vi "RT_Example.vi"() -> ()   [LabVIEW 2014]
uses:
  <vilib>/NI/cRIO Wfm/ChannelConfig.ctl
  <vilib>/FPGAPlugInAG/sbRIO-9651/niLvFpga_Open_sbRIO-9651.vi
  <vilib>/rvi/interface/common/dynamic/niFpgaDynamicAddResources.vi
  <vilib>/FPGAPlugInAG/Dynamic/niLvFpga_Reset_Dynamic.vi
  <vilib>/FPGAPlugInAG/Dynamic/niLvFpga_Run_Dynamic.vi
  <vilib>/NI/cRIO Wfm/AcqRead(Wfm).vi
  <vilib>/measure/matone.llb/Extract Single Tone Information 1 Chan.vi
  <vilib>/FPGAPlugInAG/Dynamic/niLvFpga_Close_Dynamic.vi
  <vilib>/rvi/interface/nirviOpenFPGA/nirviOpenFPGA.xnode
  FPGA Bitfiles/FPGAMainScripted.lvbitx
  <vilib>/rvi/interface/nirviMethod/nirviMethod.xnode
  <vilib>/rvi/interface/nirviCloseFPGA/nirviCloseFPGA.xnode
  <vilib>/NI/cRIO Wfm/cRIO Wfm.lvlib
  <vilib>/measure/NI_MAPro.lvlib
  <vilib>/rvi/interface/nirviReadWriteControl/nirviReadWriteControl.xnode
  NiFpgaLv.dll
  <vilib>/Utility/error.llb/Error Cluster From Error Code.vi
  <vilib>/rvi/interface/Simulation/niFpgaSimulationCallBeginRW.vi
  <vilib>/rvi/errors/niLvFpgaAdjustHostInterfaceError.vi
panel:
  out "Samples Remaining":u32
  out "Detected Amplitude (V)":dbl format="%.2p"
  out "Detected Frequency (Hz)":dbl format="%.2p"
  in  "Samples per Channel":i32=1000
  in  "Sampling Rate":u32=10000
  out "Waveform Graph":waveform(sgl)(graph)
  in  "stop":bool
  in  "Channel Info":T1=[{"Channel Name"="ai1", "Sensitivity mV_EU"=1000.0, "EU"="V", "dB Ref EU"=1.0}] {"dB Ref EU" format="%#.2p"; "Sensitivity mV_EU" format="%.2f"}
  # "Configuration Settings"
  # "Analysis"
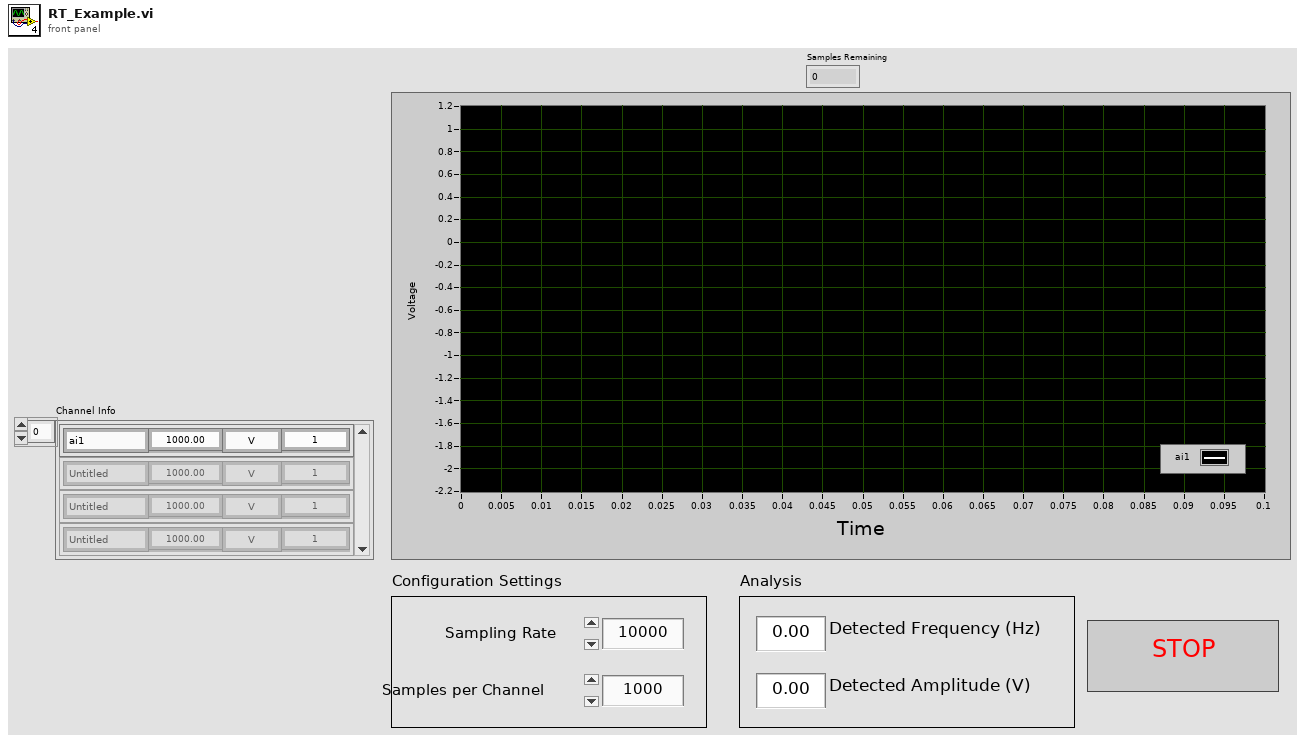
[diagram p1: front panel]
types:
  T1 = typedef "cRIO Wfm.lvlib/ChannelConfig.ctl" = cluster{"Channel Name":string, "Sensitivity mV_EU":dbl, "EU":string, "dB Ref EU":dbl}[]
  T2 = typedef "cRIO Wfm.lvlib/SamplingInfo.ctl" = cluster{"Number of Channels":i32, "Actual Samp Rate":dbl, "Chan Name Array":string[], "EU Chan Array":string[], "dB Ref Chan Array":dbl[]}
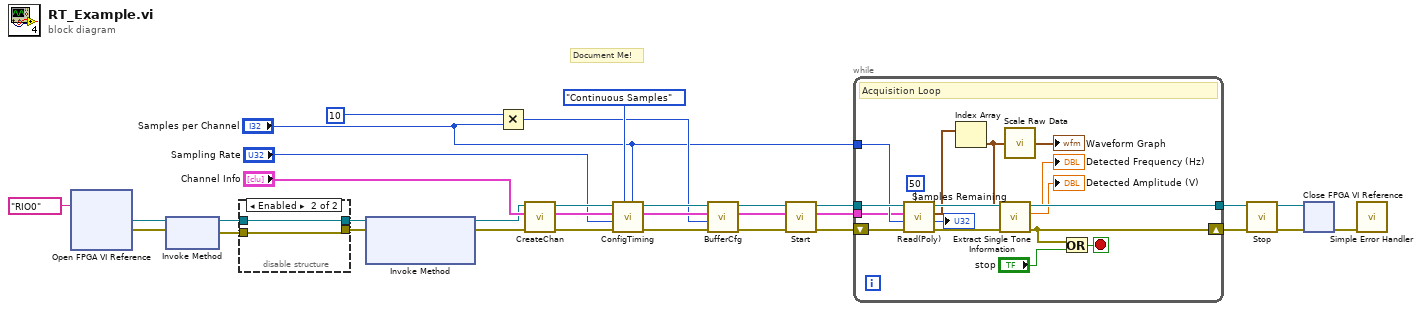
[diagram p0: block diagram]
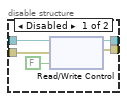
[diagram p2: hidden frame]
diagram:
  # "Document Me!"
  n1 = xnode "Open FPGA VI Reference"("resource name"=tag "RIO0") -> ("FPGA VI Reference Out"=w32:refnum<k20>, "error out"=w31:errorcluster)  [unwired: 1 in]
  n2 = xnode "Invoke Method"("FPGA VI Reference In"=w32, "error in"=w31) -> ("FPGA VI Reference Out"=w4:refnum<k20>, "error out"=w3:errorcluster)
  n3 = disable-structure shown="Enabled" {
    disable-tunnel: w4 -> [w36 w39]
    disable-tunnel: w3 -> [w35 w38]
    disable-tunnel: [w34 w39] -> w2
    disable-tunnel: [w33 w38] -> w1
    frame Disabled {
      n4 = xnode "Read/Write Control"("FPGA VI Reference In"=w36, "error in"=w35, "Debug"=FALSE) -> ("FPGA VI Reference Out"=w34:refnum<k20>, "error out"=w33:errorcluster)
    }
    frame Enabled {
    }
  }
  n5 = xnode "Invoke Method"("FPGA VI Reference In"=w2, "error in"=w1) -> ("FPGA VI Reference Out"=w5:refnum<k20>, "error out"=w6:errorcluster)  [unwired: 1 in]
  n6 = Multiply(x=10 ("y"), y="Samples per Channel") -> (x*y=w14:i32)
  n7 = call <vilib>:"CreateChan.vi"("error in"=w6, "Channel Info"="Channel Info", "Dynamic FPGA Ref"=w5) -> ("error out"=w28:errorcluster, "Sampling Info"=w27:T2, "Dynamic FPGA Ref Out"=w30:refnum<k20>)  [unwired: 6 in]
  n8 = call <vilib>:"ConfigTiming.vi"("Samples per Channel"="Samples per Channel", "Sample Mode"=enum16{"Finite Samples", "Continuous Samples"}."Continuous Samples", "error in"=w28, "Sample Rate"="Sampling Rate", "Sampling Info In"=w27, "Dynamic FPGA Ref"=w30) -> ("error out"=w25:errorcluster, "Sampling Info Out"=w24:T2, "Dynamic FPGA Ref Out"=w26:refnum<k20>)  [unwired: 2 in, 1 out]
  n9 = call <vilib>:"BufferCfg.vi"("error in"=w25, "Buffer Size [Samps per Chan]"=w14, "Sampling Info In"=w24, "Dynamic FPGA Ref"=w26) -> ("error out"=w22:errorcluster, "Sampling Info Out"=w21:T2, "Dynamic FPGA Ref Out"=w23:refnum<k20>)  [unwired: 4 in, 1 out]
  n10 = call <vilib>:"Start.vi"("error in"=w22, "Sampling Info In"=w21, "Dynamic FPGA Ref"=w23) -> ("error out"=w8:errorcluster, "Sampling Info Out"=w11:T2, "Dynamic FPGA Ref Out"=w9:refnum<k20>)  [unwired: 6 in]
  n11 = while {
    tunnel: w9 -> [w55]
    shift-right: [w43] -> w18
    shift-left: w8 -> [w54]
    tunnel: [w53] -> w17
    tunnel: "Samples per Channel" -> [w52]
    tunnel: w11 -> [w51]
    stop <- w44 stop-if-true
    # "Acquisition Loop"
    n12 = call-poly <vilib>:"Read(Poly).vi"("Poll Time (ms)"=u32 50, "error in"=w54, "Samps Read per Chan"=w52, "Sampling Info"=w51, "Dynamic FPGA Ref"=w55) -> ("error out"=w47:errorcluster, "Samples Remaining"=→"Samples Remaining":u32, "Wfm Data"=w42:waveform(sgl)[], "Dynamic FPGA Ref Out"=w53:refnum<k20>)  [unwired: 3 in]
    n13 = Index Array(array=w42) -> (element=w41:waveform(sgl))  [unwired: 1 in]
    n14 = call-poly <vilib>:"Extract Single Tone Information.vi"("error in (no error)"=w47, "time signal in"=w41) -> ("error out"=w43:errorcluster, "detected amplitude"=→"Detected Amplitude (V)":dbl, "detected frequency"=→"Detected Frequency (Hz)":dbl)  [unwired: 4 in, 3 out]
    n15 = call "Scale Raw Data.vi"("Waveform in"=w41) -> ("Waveform out"=→"Waveform Graph":waveform(sgl))  [unwired: 14 in]
    n16 = Or(x=w43, y="stop") -> (x .or. y?=w44:bool)
  }
  n17 = call <vilib>:"Stop.vi"("error in"=w18, "Dynamic FPGA Ref"=w17) -> ("error out"=w15:errorcluster, "Dynamic FPGA Ref Out"=w16:refnum<k20>)  [unwired: 8 in]
  n18 = xnode "Close FPGA VI Reference"("FPGA VI Reference In"=w16, "error in"=w15) -> ("error out"=w7:errorcluster)
  n19 = call <vilib>:"Simple Error Handler.vi"("error in (no error)"=w7) -> ()  [unwired: 4 in, 5 out]
